vi "Continue if it True.vi"(6 "Test":bool, 7 "i":i32, 8 "N":i32) -> (1 "Action":bool, 2 "i duplicate":i32)   [LabVIEW 2020, in "Exaprom PDF.lvlib"]
uses:
  <userlib>/labview-PDF-writer-master/Exaprom PDF.lvlib
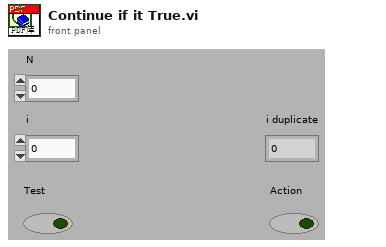
[diagram p1: front panel]
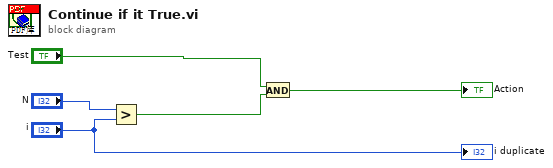
[diagram p0: block diagram]
diagram:
  n1 = Greater?(x="N", y="i") -> (0:w4:bool)
  n2 = And(x="Test", y=w4) -> (x .and. y?=→"Action":bool)
  "i duplicate" <- "i"
